vi "controlVI.vi"(8 "monitorToUse":u16, 9 "Front Panel Window:Window Bounds":T1, 10 "colors":u32[](array[numeric]), 11 "8-bit pixmap":u8[][](array[numeric])) -> (1 "projSize":i32[](array[numeric]))   [LabVIEW 2017]
uses:
  <vilib>/Utility/miscctls.llb/LVRectTypeDef.ctl
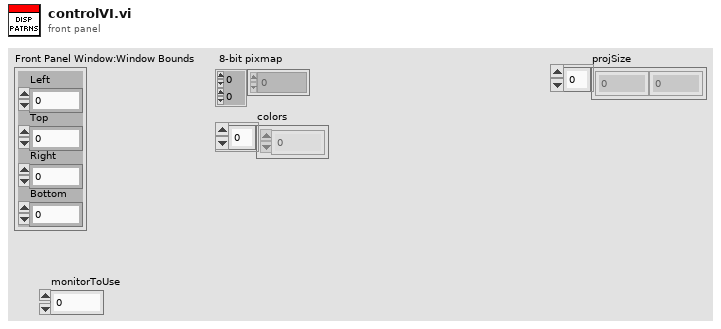
[diagram p1: front panel]
types:
  T1 = typedef "LVRectTypeDef.ctl" = cluster{"Left":i16, "Top":i16, "Right":i16, "Bottom":i16}
  T2 = enum32{"Invalid", "Standard", "Closed", "Hidden", "Minimized", "Maximized"}
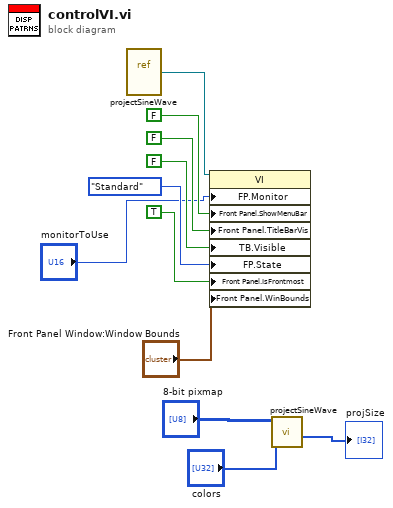
[diagram p0: block diagram]
diagram:
  n1 = vi-ref "projectSineWave.vi"() -> (w11:refnum<vi>)
  n2 = property class="VI"(reference=w11, "FP.Monitor"="monitorToUse", "Front Panel.ShowMenuBar"=FALSE ("Front Panel Window:Show Menu Bar"), "Front Panel.TitleBarVis"=FALSE ("Front Panel Window:Title Bar Visible"), "TB.Visible"=FALSE ("Tool Bar:Visible"), "FP.State"=T2."Standard" ("Front Panel Window:State"), "Front Panel.IsFrontmost"=TRUE ("Front Panel Window:Is Frontmost"), "Front Panel.WinBounds"="Front Panel Window:Window Bounds") -> ()  [unwired: 1 in, 2 out]
  n3 = call "projectSineWave.vi"("colors"="colors", "8-bit pixmap"="8-bit pixmap") -> ("projSize"=→"projSize":i32[])  [unwired: 8 in, 1 out]
